vi "Check WP position.vi"(6 "threshold":dbl, 7 "target":dbl, 8 "error in (no error)":errorcluster, 9 "recheck pos time":dbl, 10 "lChanID":i32, 11 "Automation Refnum in":refnum<k7>) -> (0 "error out":errorcluster, 2 "Current Position":sgl, 3 "Automation Refnum out":refnum<k7>)   [LabVIEW 2015]
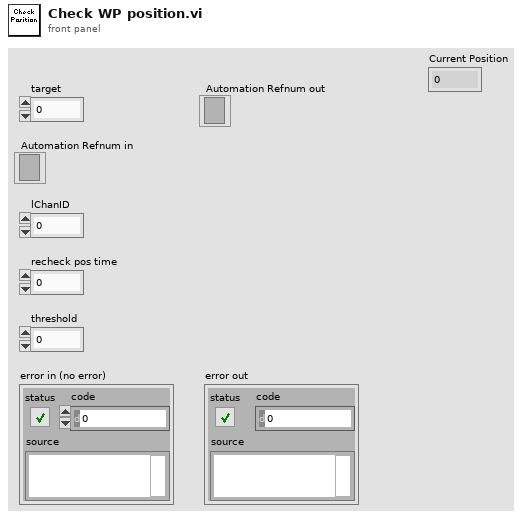
[diagram p1: front panel]
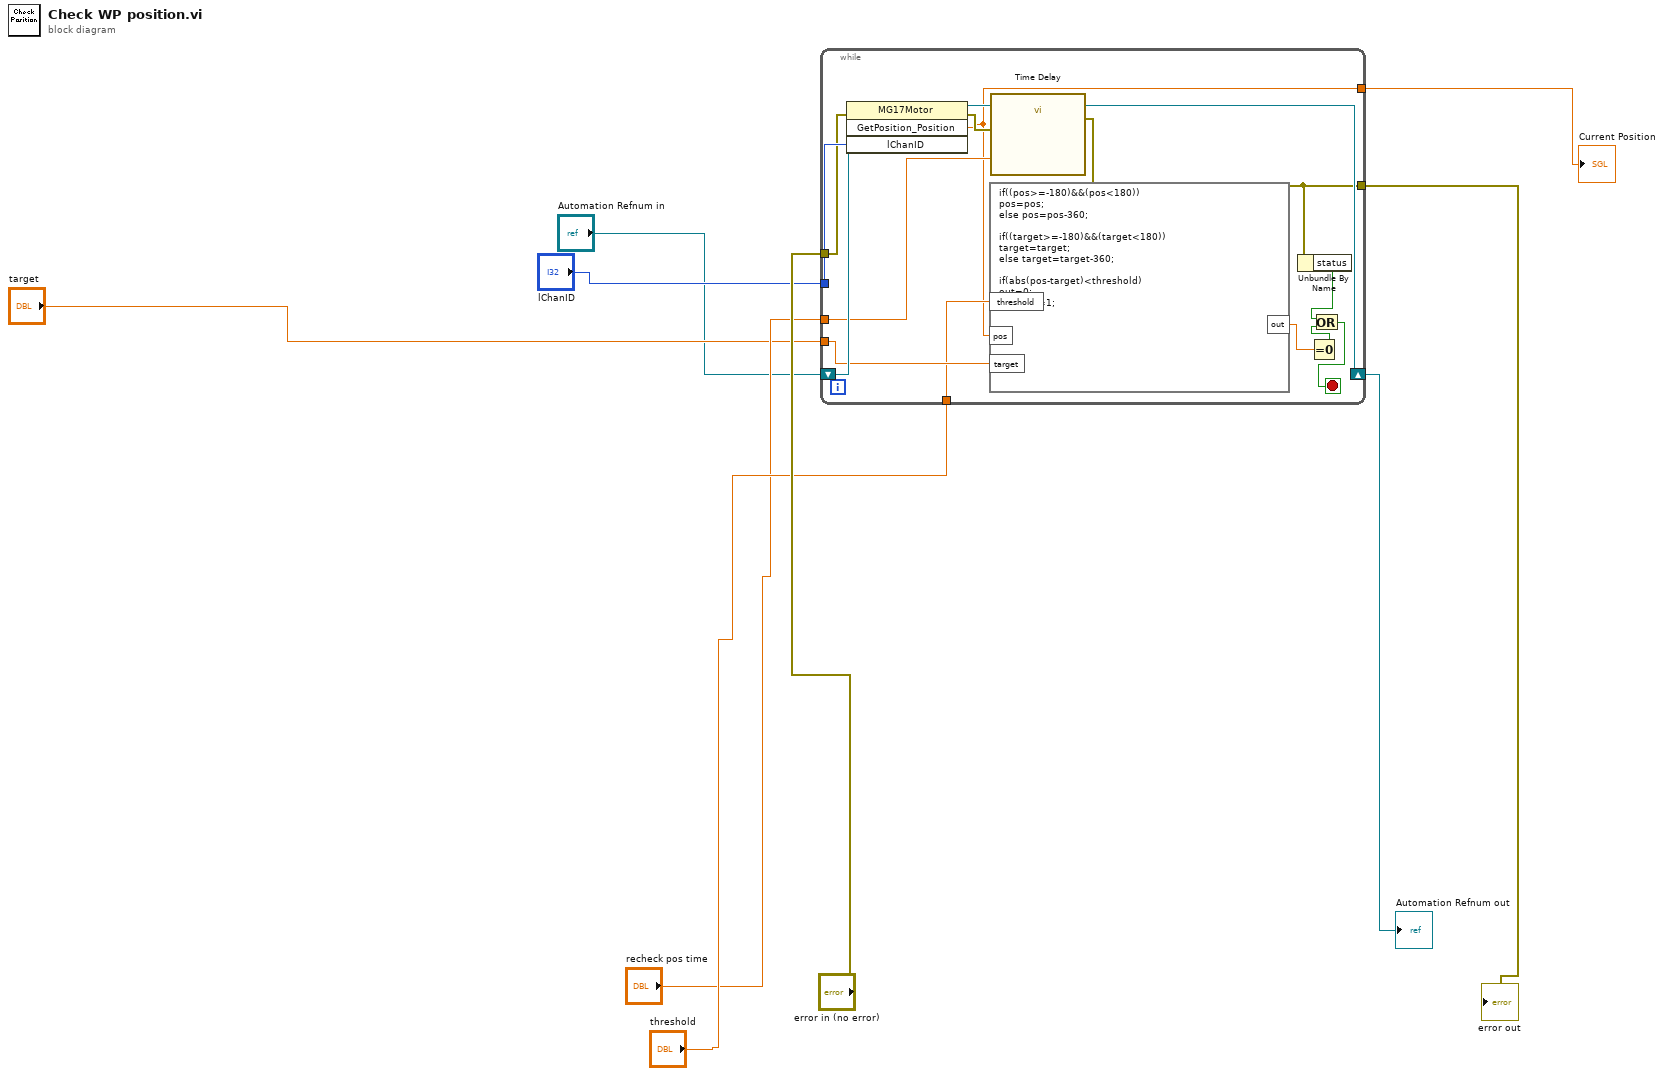
[diagram p0: block diagram]
diagram:
  n1 = while {
    tunnel: "lChanID" -> [w21]
    shift-right: [w22] -> w3
    shift-left: "Automation Refnum in" -> [w23]
    tunnel: "target" -> [w17]
    tunnel: "recheck pos time" -> [w20]
    tunnel: "threshold" -> [w16]
    tunnel: "error in (no error)" -> [w19]
    tunnel: [w13] -> w9
    tunnel: [w14] -> w1
    stop <- w10 stop-if-true
    n2 = invoke class="MG17Motor" method="GetPosition_Position"(reference=w23, error in=w19, "lChanID"=w21) -> (reference out=w22:refnum<k7>, error out=w18:errorcluster, "GetPosition_Position"=w14:sgl)  [unwired: 1 in, 1 out]
    n3 = formula code="if((pos>=-180)&&(pos<180))\npos=pos;\nelse pos=pos-360;\n\nif((target>=-180)&&(target<180))\ntarget=target;\nelse target=target-360;\n\nif(abs(pos-target)<threshold)\nout=0;\nelse out=1;"("pos"=w14, "target"=w17, "threshold"=w16) -> ("out"=w15:dbl)
    n4 = call "Time Delay"("error in (no error)"=w18, "Delay Time (s)"=w20) -> ("error out"=w13:errorcluster)  [unwired: 9 in]
    n5 = Unbundle By Name(w13) -> ("status"=w11:bool)
    n6 = Equal To 0?(x=w15) -> (x = 0?=w12:bool)
    n7 = Or(x=w11, y=w12) -> (x .or. y?=w10:bool)
  }
  "error out" <- w9
  "Automation Refnum out" <- w3
  "Current Position" <- w1
